vi "fastFrame_get_average.vi"(4 "array":dbl[][](array[numeric]), 5 "fast frame count":i32) -> (0 "averaged molecular frames":dbl[](array[numeric]), 2 "averaged background frames":dbl[](array[numeric]))   [LabVIEW 2011]
doc: "This Vi averages the frames for both the background and the molecular cycle and subtracts the background from the molecular signal in the time domain"
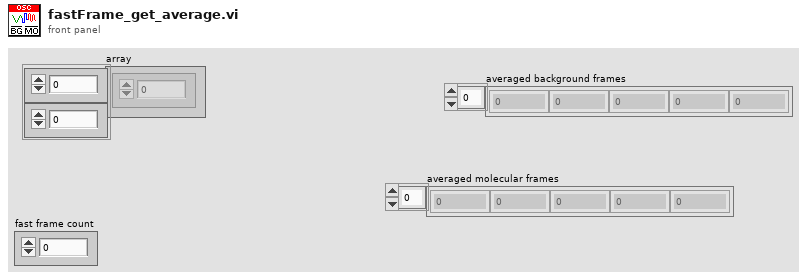
[diagram p1: front panel]
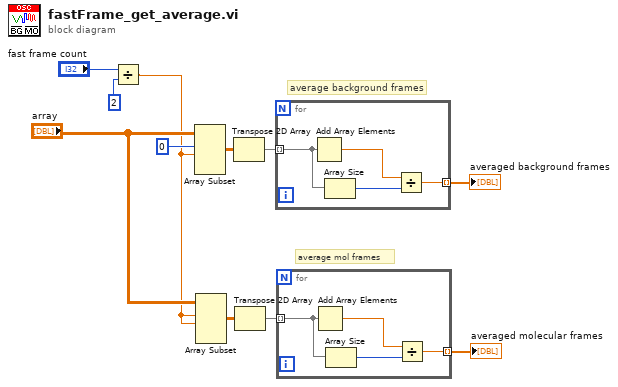
[diagram p0: block diagram]
diagram:
  # "average mol frames"
  # "average background frames"
  n1 = Divide(x="fast frame count", y=2 ("x")) -> (x/y=w1:dbl)
  n2 = Array Subset(array="array", index (row)=0 ("index"), length (row)=w1) -> (w6:dbl[][])  [unwired: 2 in]
  n3 = Array Subset(array="array", index (row)=w1, length (row)=w1) -> (w3:dbl[][])  [unwired: 2 in]
  n4 = Transpose 2D Array(2D array=w6) -> (transposed array=w8:dbl[][])
  n5 = Transpose 2D Array(2D array=w3) -> (transposed array=w5:dbl[][])
  n6 = for {
    tunnel: w8 -> [w13] mode=indexing
    tunnel: [w14] -> w7 mode=indexing
    n7 = Add Array Elements(numeric array=w13) -> (sum=w15:dbl)
    n8 = Array Size(array=w13) -> (size(s)=w12:i32)
    n9 = Divide(x=w15, y=w12) -> (x/y=w14:dbl)
  }
  "averaged background frames" <- w7
  n10 = for {
    tunnel: w5 -> [w17] mode=indexing
    tunnel: [w18] -> w4 mode=indexing
    n11 = Add Array Elements(numeric array=w17) -> (sum=w19:dbl)
    n12 = Array Size(array=w17) -> (size(s)=w16:i32)
    n13 = Divide(x=w19, y=w16) -> (x/y=w18:dbl)
  }
  "averaged molecular frames" <- w4
